vi "GenerateProjectPath.vi"(9 "Device Code":u32, 10 "Project Name":string, 11 "Location Path":path) -> (3 "Project Path":path)   [LabVIEW 2021, in "myRIOMetaDataObj.lvclass"]
uses:
  myRIOMetaDataObj.lvclass
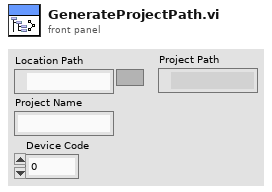
[diagram p1: front panel]
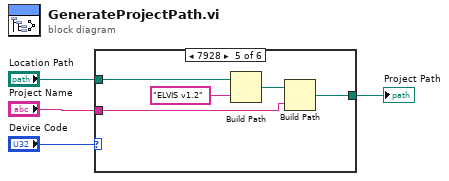
[diagram p0: block diagram]
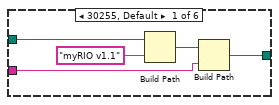
[diagram p2: hidden frame]
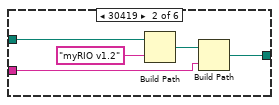
[diagram p3: hidden frame]
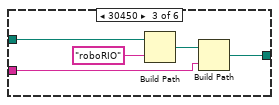
[diagram p4: hidden frame]
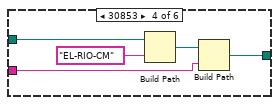
[diagram p5: hidden frame]
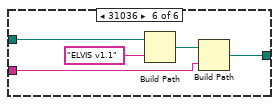
[diagram p6: hidden frame]
diagram:
  n1 = case shown="7928" "Device Code" {
    tunnel: "Location Path" -> [w9 w14 w19 w24 w29 w34]
    tunnel: [w5 w10 w15 w20 w25 w30] -> w3
    tunnel: "Project Name" -> [w6 w11 w16 w21 w26 w31]
    frame 30255, Default {
      n2 = Build Path(base path=w9, name or relative path="myRIO v1.1") -> (appended path=w7:path)
      n3 = Build Path(base path=w7, name or relative path=w6) -> (appended path=w5:path)
    }
    frame 30419 {
      n4 = Build Path(base path=w14, name or relative path="myRIO v1.2") -> (appended path=w12:path)
      n5 = Build Path(base path=w12, name or relative path=w11) -> (appended path=w10:path)
    }
    frame 30450 {
      n6 = Build Path(base path=w19, name or relative path="roboRIO") -> (appended path=w17:path)
      n7 = Build Path(base path=w17, name or relative path=w16) -> (appended path=w15:path)
    }
    frame 30853 {
      n8 = Build Path(base path=w24, name or relative path="EL-RIO-CM") -> (appended path=w22:path)
      n9 = Build Path(base path=w22, name or relative path=w21) -> (appended path=w20:path)
    }
    frame 31016 {
      n10 = Build Path(base path=w29, name or relative path="ELVIS v1.2") -> (appended path=w27:path)
      n11 = Build Path(base path=w27, name or relative path=w26) -> (appended path=w25:path)
    }
    frame 31036 {
      n12 = Build Path(base path=w34, name or relative path="ELVIS v1.1") -> (appended path=w32:path)
      n13 = Build Path(base path=w32, name or relative path=w31) -> (appended path=w30:path)
    }
  }
  "Project Path" <- w3
